vi "LockStartEndLine.vi"(10 "index":i32, 11 "All Lines":T1) -> (3 "Not Locked?":bool)   [LabVIEW 2014]
uses:
  Libraries/Map Data Folder/All-Lines.ctl
  Libraries/Map Data Folder/LineCluster.ctl
  Libraries/Map Data Folder/LineConnection.ctl
  Libraries/Map Data Folder/Map Data.lvlib
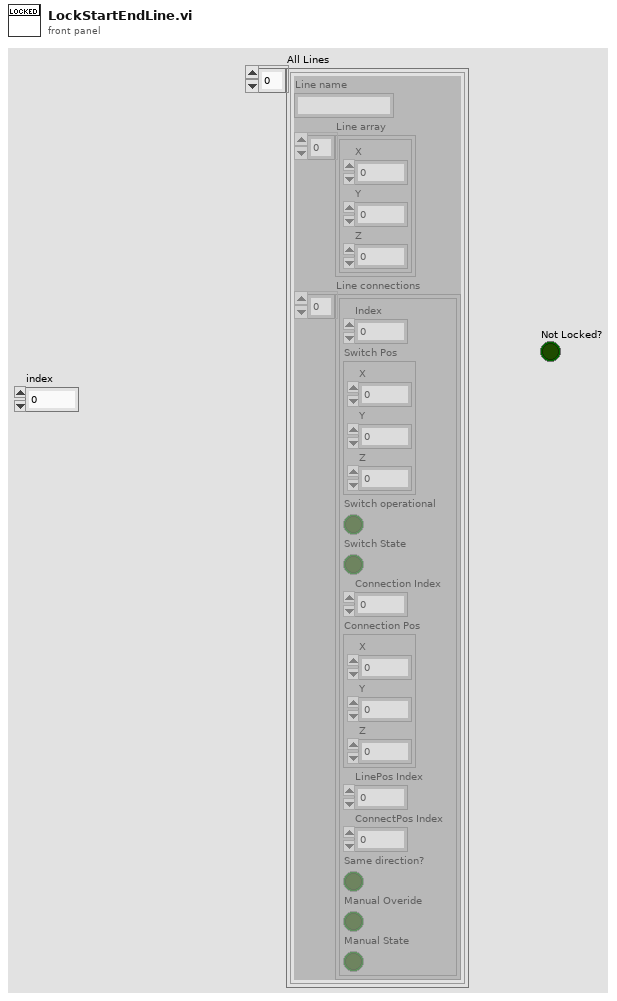
[diagram p1: front panel]
types:
  T1 = typedef "Map Data.lvlib/All-Lines.ctl" = T2[]
  T2 = typedef "Map Data.lvlib/LineCluster.ctl" = cluster{"Line name":string, "Line array":cluster{"X":dbl, "Y":dbl, "Z":dbl}[], "Line connections":T3[]}
  T3 = typedef "LineConnection.ctl" = cluster{"Index":i32, "Switch Pos":cluster{"X":dbl, "Y":dbl, "Z":dbl}, "Switch operational":bool, "Switch State":bool, "Connection Index":i32, "Connection Pos":cluster{"X":dbl, "Y":dbl, "Z":dbl}, "LinePos Index":i32, "ConnectPos Index":i32, "Same direction?":bool, "Manual Overide":bool, "Manual State":bool}
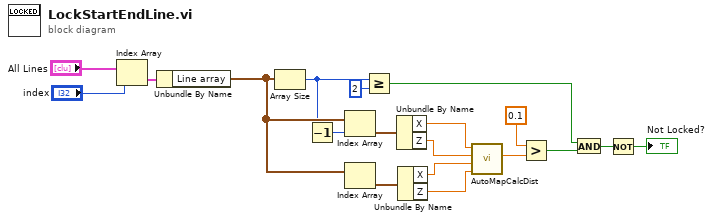
[diagram p0: block diagram]
diagram:
  n1 = Index Array(array="All Lines", index="index") -> (element=w17:T2)
  n2 = Unbundle By Name(w17) -> ("Line array"=w16:cluster{"X":dbl, "Y":dbl, "Z":dbl}[])
  n3 = Array Size(array=w16) -> (size(s)=w5:i32)
  n4 = Decrement(x=w5) -> (x-1=w15:i32)
  n5 = Index Array(array=w16, index=w15) -> (element=w14:cluster{"X":dbl, "Y":dbl, "Z":dbl})
  n6 = Index Array(array=w16) -> (element=w13:cluster{"X":dbl, "Y":dbl, "Z":dbl})  [unwired: 1 in]
  n7 = Greater Or Equal?(x=w5, y=2) -> (x >= y?=w2:bool)
  n8 = Unbundle By Name(w14) -> ("X"=w10:dbl, "Z"=w9:dbl)
  n9 = Unbundle By Name(w13) -> ("X"=w12:dbl, "Z"=w11:dbl)
  n10 = call "AutoMapCalcDist.vi"("Y2"=w11, "X2"=w12, "Y1"=w9, "X1"=w10) -> ("Distance"=w7:dbl)  [unwired: 7 in]
  n11 = Greater?(x=0.1, y=w7) -> (0:w6:bool)
  n12 = And(x=w2, y=w6) -> (x .and. y?=w3:bool)
  n13 = Not(x=w3) -> (.not. x?=→"Not Locked?":bool)
